vi "PH_Tektronix_7000.Revision.vi"(0 "i ref in":refnum<vi>, 5 "error IO":errorcluster) -> (14 "i ref out":refnum<vi>, 19 "error out":errorcluster)   [LabVIEW 2014, in "PH_Tektronix_7000.lvlib"]
doc: "If the connection is established, this VI queries the instrumnent driver revision, the instrument firmware revision, and errors which are written to own attributes."
uses:
  PH_Tektronix_7000.lvlib
  instr.lib/Tektronix7000Series/Tektronix 7000 Series - Driver np.lvlib
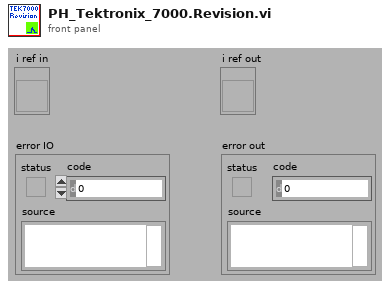
[diagram p1: front panel]
types:
  T1 = typedef "PH_Tektronix_7000.lvlib/PH_Tektronix_7000.i attribute.ctl" = cluster{"VISA Resource Name":refnum<visa-resource-name>, "IDN":cluster{"Instrument Driver":string, "Instrument Firmware":string, "Model":string, "Serial Number":string}, "Selftest":cluster{"Result":i32, "Message":string}, "Trigger Configuration":T2, "Acquisition Configuration":T3, "GUI Refs":T4, "State":T5, "Error Message":string, "Allow Prdc Loop?":bool, "Channel 1":T6, "Channel 2":T6, "Channel 3":T6, "Channel 4":T6, "Data CH 1":waveform(dbl), "Data CH 2":waveform(dbl), "Data CH 3":waveform(dbl), "Data CH 4":waveform(dbl), "Allow config?":bool, "Name Channel 1":string, "Name Channel 2":string, "Name Channel 3":string, "Name Channel 4":string, "Fetch Data before sending to PSDB?":bool, "Constructor passed?":bool, "Data taken at":timestamp, "Plot Colors":u32[], "Default VISA Resource":string}
  T2 = typedef "PH_Tektronix_7000.lvlib/PH_Tektronix_7000.Trigger Config.ctl" = cluster{"Source":u16, "Level [V]":dbl, "Slope":u16, "Coupling":u16, "Trigger Mode":u16}
  T3 = typedef "PH_Tektronix_7000.lvlib/PH_Tektronix_7000.Acquisition Config.ctl" = cluster{"Record Length":u32, "Timebase [s/div]":dbl, "Position [%]":dbl, "Acquisition Type":u16, "Average Waveforms":i32, "Envelope Waveforms":i32, "WfmDB Samples":i32, "Continuous?":bool, "Delay [s]":dbl, "Run?":bool}
  T4 = typedef "PH_Tektronix_7000.lvlib/PH_Tektronix_7000.GUI Refs.ctl" = cluster{"Graph":refnum<vi>, "State":refnum<vi>, "Delete":refnum<vi>, "VISA Resource":refnum<vi>, "Allow Configure":refnum<vi>, "Fetch Data":refnum<vi>, "Fetch before sending Data to PSDB":refnum<vi>, "Name Channel 1":refnum<vi>, "Name Channel 2":refnum<vi>, "Name Channel 3":refnum<vi>, "Name Channel 4":refnum<vi>, "Prdc Intervall [ms]":refnum<vi>, "Data taken":refnum<vi>, "Model":refnum<vi>, "Serial Number":refnum<vi>, "Firmware":refnum<vi>, "Driver":refnum<vi>, "Acquisition":refnum<vi>, "Trigger":refnum<vi>, "Cursor: D Time [s]":refnum<vi>, "Cursor: D Signal [V]":refnum<vi>, "Channel 1":refnum<vi>, "Channel 2":refnum<vi>, "Channel 3":refnum<vi>, "Channel 4":refnum<vi>}
  T5 = typedef "PH_StatusHandler.lvlib/PH_StatusHandler.Status.ctl" = i16
  T6 = typedef "PH_Tektronix_7000.lvlib/PH_Tektronix_7000.Channel Config.ctl" = cluster{"Enable Channel":bool, "Bandwidth":u16, "Input Impedance":u16, "Vertical Coupling":u16, "Probe Attenuation":dbl, "Range [V/div]":dbl, "Position [div]":dbl, "Bandwidth raw":string}
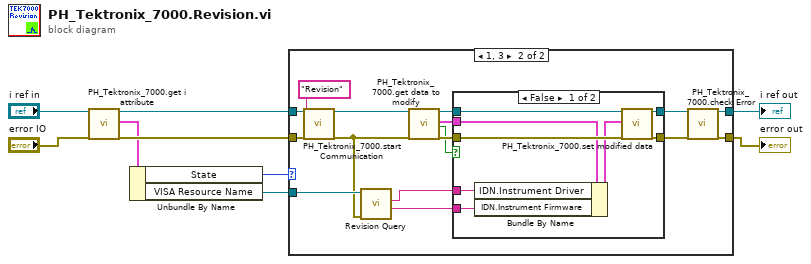
[diagram p0: block diagram]
diagram:
  n1 = call "PH_Tektronix_7000.get i attribute.vi"("i ref in"="i ref in", "error in (no error)"="error IO") -> ("i ref out"=w3:refnum<vi>, "i attribute"=w5:T1, "error out"=w7:errorcluster)  [unwired: 15 in]
  n2 = Unbundle By Name(w5) -> ("State"=w9:T5, "VISA Resource Name"=w6:refnum<visa-resource-name>)
  n3 = case shown="1, 3" w9 {
    tunnel: w3 -> [w11 w13]
    tunnel: w6 -> [_ w22]
    tunnel: w7 -> [w10 w21]
    tunnel: [w11 w17] -> w8
    tunnel: [w10 w15] -> w1
    frame Default {
    }
    frame 1, 3 {
      n4 = call "PH_Tektronix_7000.start Communication.vi"("i ref in"=w13, "Action"="Revision", "error in"=w21) -> ("i ref out"=w14:refnum<vi>, "error out"=w18:errorcluster)  [unwired: 15 in]
      n5 = call "Revision Query.vi"("error in (no error)"=w18, "VISA resource name"=w22) -> ("Instrument Firmware Revision"=w19:string, "Instrument Driver Revision"=w20:string)  [unwired: 6 in, 2 out]
      n6 = call "PH_Tektronix_7000.get data to modify.vi"("i ref in"=w14, "error in (no error)"=w18) -> ("i ref out"=w25:refnum<vi>, "i attribute"=w23:T1, "timed out"=w24:bool, "error out"=w26:errorcluster)  [unwired: 14 in]
      n7 = case shown="False" w24 {
        tunnel: [w35 w36] -> w16
        tunnel: w26 -> [w34 w36]
        tunnel: w25 -> [w33 w37]
        tunnel: [w32 w37] -> w27
        tunnel: w23 -> [w31 _]
        tunnel: w20 -> [w29 _]
        tunnel: w19 -> [w28 _]
        frame False {
          n8 = Bundle By Name(cluster=w31, "IDN.Instrument Driver"=w29, "IDN.Instrument Firmware"=w28) -> (w30:T1)
          n9 = call "PH_Tektronix_7000.set modified data.vi"("i ref in"=w33, "i attribute"=w30, "error in (no error)"=w34) -> ("i ref out"=w32:refnum<vi>, "error out"=w35:errorcluster)  [unwired: 15 in]
        }
        frame True {
        }
      }
      n10 = call "PH_Tektronix_7000.check Error.vi"("i ref in"=w27, "error in"=w16) -> ("i ref out"=w17:refnum<vi>, "error out"=w15:errorcluster)  [unwired: 16 in]
    }
  }
  "i ref out" <- w8
  "error out" <- w1
